vi "Detect Multiple (Greyscale).vi"(8 "error in (no error)":errorcluster, 10 "Greyscale Image in":T3, 11 "QR Code Detector in":refnum<class "QR Code Detector.lvclass">) -> (0 "error out":errorcluster, 1 "Detections":T1[](array[typedef]), 2 "Greyscale Image":T3, 3 "QR Code Detector":refnum<class "QR Code Detector.lvclass">, 4 "Number of Detections":i32)   [LabVIEW 2020, in "feature_detection.lvlib" / "QR Code Detector.lvclass"]
doc: "Detect multiple QR Codes in an image."
uses:
  QR Code Detector.lvclass
  image/Greyscale Image.ctl
  common/Image Points Quad (Float).ctl
  common/Image Point (Float).ctl
  QR Code Detector.lvclass/QR Code Detector.ctl
  a11a4014-6d36-4b83-8619-6a5cddee6c3f.vi
  <vilib>/Utility/error.llb/Error Cluster From Error Code.vi
  common/common.lvlib
  image/image.lvlib
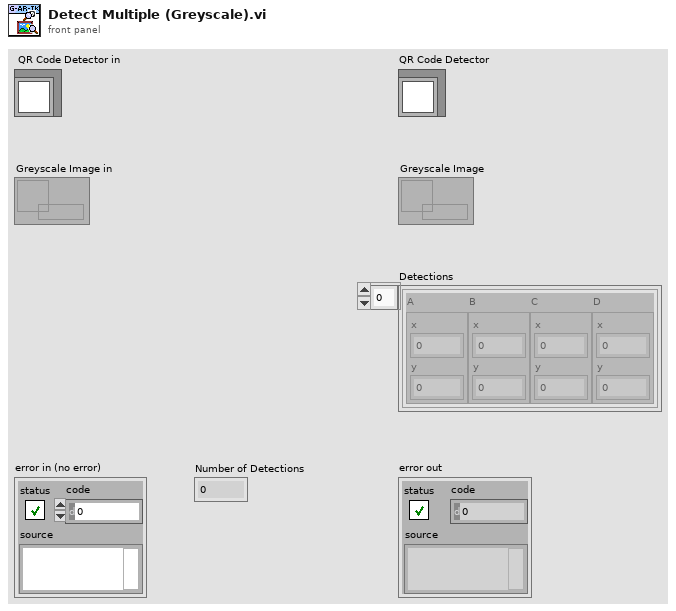
[diagram p1: front panel]
types:
  T1 = typedef "common.lvlib/Image Points Quad (Float).ctl" = cluster{"A":T2, "B":T2, "C":T2, "D":T2}
  T2 = typedef "common.lvlib/Image Point (Float).ctl" = cluster{"x":dbl, "y":dbl}
  T3 = typedef "image.lvlib/Greyscale Image.ctl" = refnum<data-value>
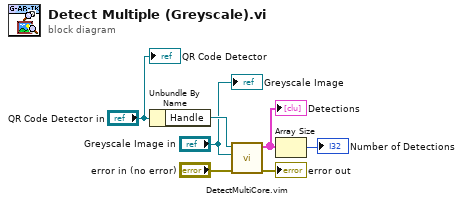
[diagram p0: block diagram]
diagram:
  n1 = Unbundle By Name("QR Code Detector in") -> ("Handle"=w5:refnum<data-value>)
  n2 = call "DetectMultiCore.vim"("error in (no error)"="error in (no error)", "Greyscale Image"="Greyscale Image in", "Handle"=w5) -> ("error out"=→"error out":errorcluster, "Detections"=w1:T1[])  [unwired: 7 in]
  "Detections" <- w1
  n3 = Array Size(array=w1) -> (size(s)=→"Number of Detections":i32)
  "QR Code Detector" <- "QR Code Detector in"
  "Greyscale Image" <- "Greyscale Image in"
